vi "VBSArmOrStop.vi"(3 "error in (no error)":errorcluster, 4 "Arm T/Stop F":bool, 5 "ActXDSO In":refnum<k7>) -> (0 "error out":errorcluster, 2 "ActXDSO Out":refnum<k7>)   [LabVIEW 2022 SP3]
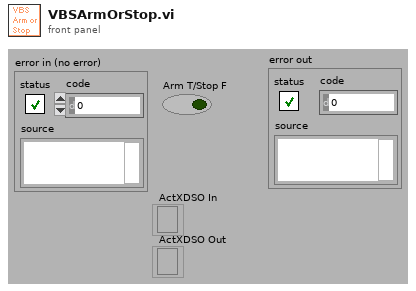
[diagram p1: front panel]
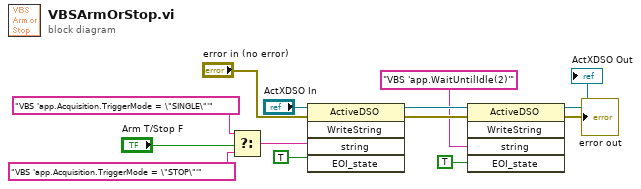
[diagram p0: block diagram]
diagram:
  n1 = Select(t="VBS 'app.Acquisition.TriggerMode = \"SINGLE\"'", s="Arm T/Stop F", f="VBS 'app.Acquisition.TriggerMode = \"STOP\"'") -> (s? t:f=w10:string)
  n2 = invoke class="ActiveDSO" method="WriteString"(reference="ActXDSO In", error in="error in (no error)", "string"=w10, "EOI_state"=TRUE) -> (reference out=w6:refnum<k7>, error out=w5:errorcluster)  [unwired: 1 in, 3 out]
  n3 = invoke class="ActiveDSO" method="WriteString"(reference=w6, error in=w5, "string"="VBS 'app.WaitUntilIdle(2)'", "EOI_state"=TRUE) -> (reference out=→"ActXDSO Out":refnum<k7>, error out=→"error out":errorcluster)  [unwired: 1 in, 3 out]
